vi "Extract TDMS FGEN Info.vi"(8 "error in (no error)":errorcluster, 10 "TDMS Name Mapping":T1, 11 "TDMS File Path":path) -> (0 "error out":errorcluster, 1 "FGEN Sample Rate":dbl, 2 "FGEN Wfm Map":map{string, waveform(dbl)[]}(c390), 3 "FGEN Channels":string[](array[string]), 4 "Gain Per Channel":dbl[](array[numeric]))   [LabVIEW 2025]
uses:
  <vilib>/ErrorRing/Error Ring.xnode
  <vilib>/Utility/error.llb/Error Cluster From Error Code.vi
  Typedef/TDMS Name Mapping.ctl
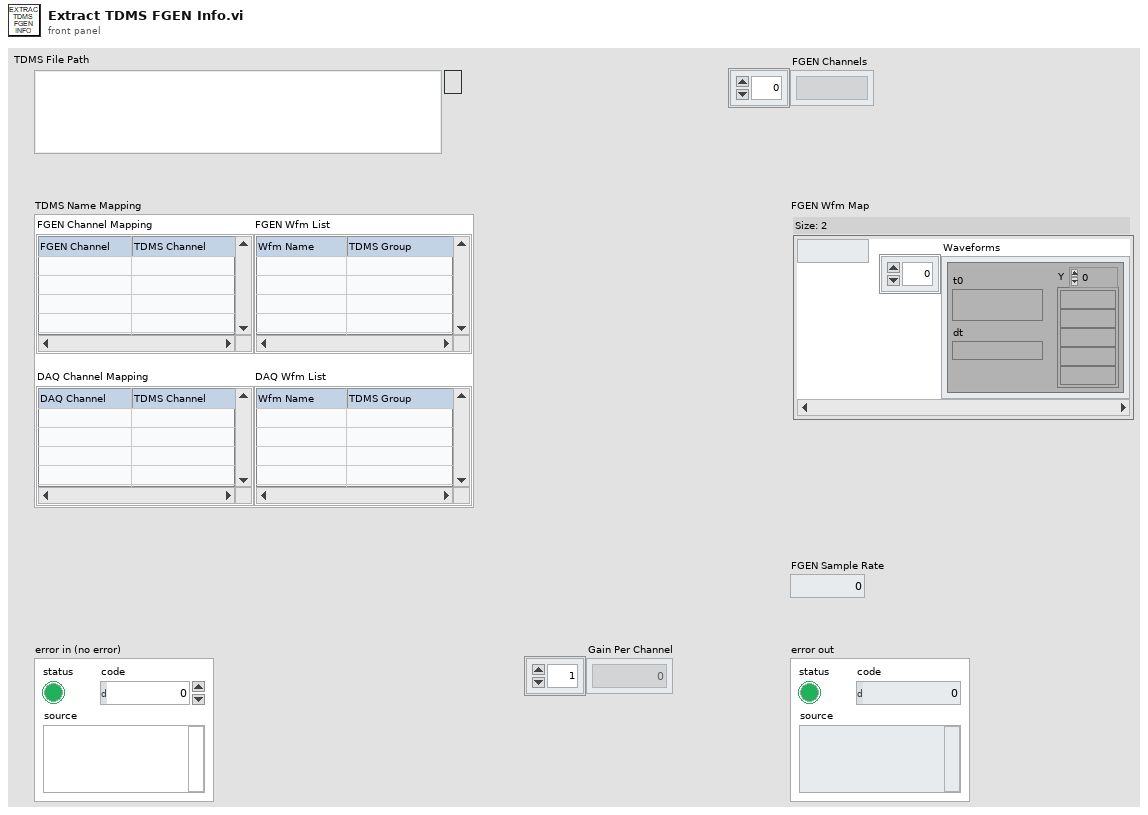
[diagram p1: front panel]
types:
  T1 = typedef "TDMS Name Mapping.ctl" = cluster{"FGEN Channel Mapping":string[][], "DAQ Channel Mapping":string[][], "FGEN Wfm List":string[][], "DAQ Wfm List":string[][]}
  T2 = enum16{"open", "open or create", "create or replace", "create", "open (read-only)"}
  T3 = enum16{"Error or Wfm Not Found", "Not all Chns Found", "All Found"}
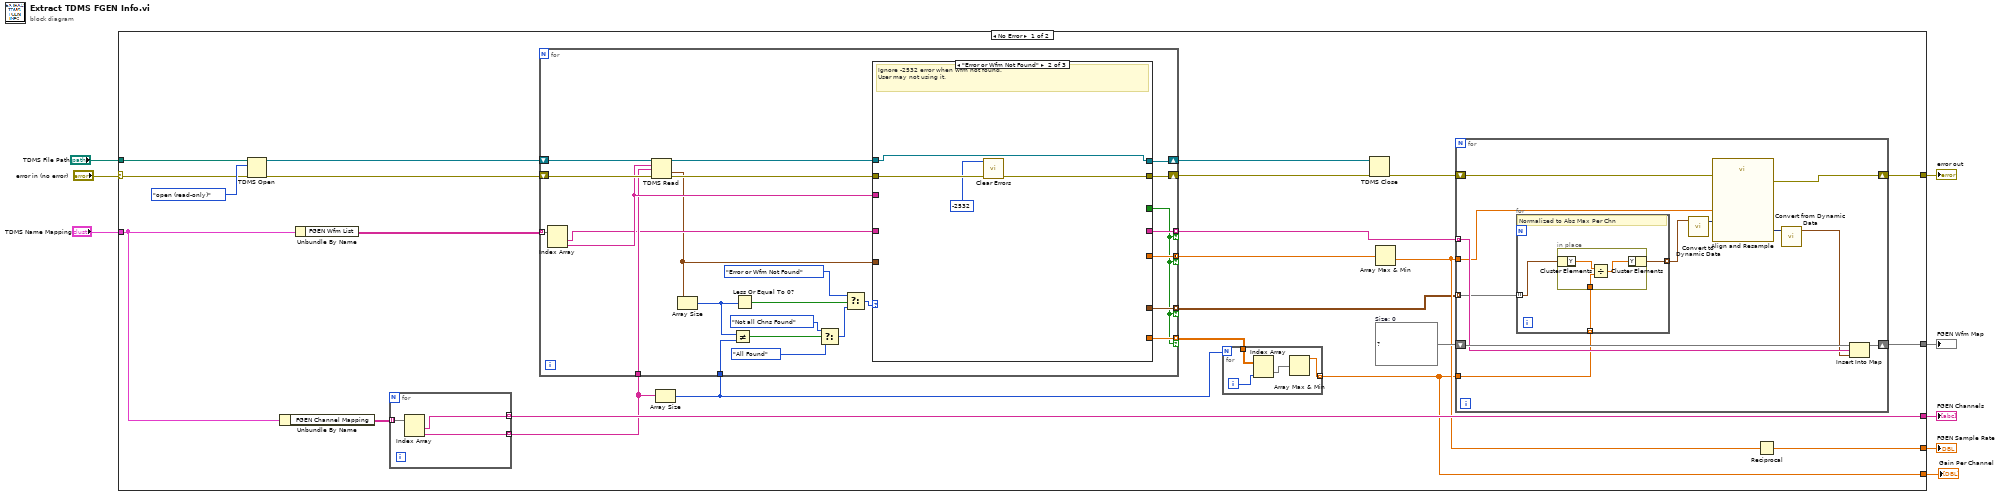
[diagram p0: block diagram]
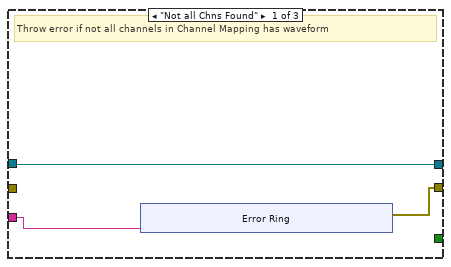
[diagram p2: hidden frame]
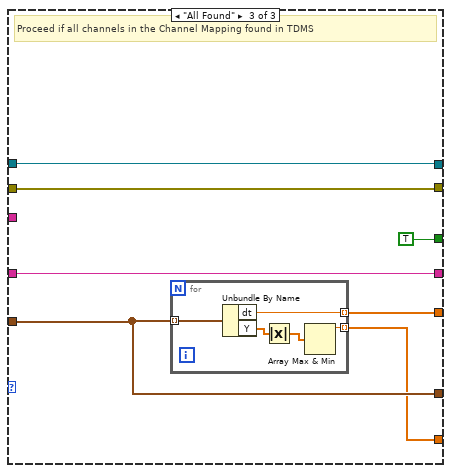
[diagram p3: hidden frame]
diagram:
  n1 = case shown="No Error" "error in (no error)" {
    selector: "error in (no error)" -> [w23 w109]
    tunnel: "TDMS File Path" -> [w30 _]
    tunnel: [w29 _] -> w7
    tunnel: [w18 w109] -> w6
    tunnel: [w17 _] -> w4
    tunnel: [w15 _] -> w3
    tunnel: "TDMS Name Mapping" -> [w13 _]
    tunnel: [w9 _] -> w1
    frame No Error {
      w21 = map{string, waveform(dbl)[]} {}  # Size: 0
      n2 = TDMS Open(8:w23, 10:T2."open (read-only)" ("operation (0:open)"), 11:w30) -> (0:w27:errorcluster, 3:w28:refnum<k34>)  [unwired: 4 in]
      n3 = Unbundle By Name(w13) -> ("FGEN Channel Mapping"=w31:string[][])
      n4 = Unbundle By Name(w13) -> ("FGEN Wfm List"=w32:string[][])
      n5 = for {
        tunnel: w31 -> [w39] mode=indexing
        tunnel: [w38] -> w29 mode=indexing
        tunnel: [w37] -> w14 mode=indexing
        n6 = Index Array(array=w39) -> (element #1=w38:string, element #2=w37:string)  [unwired: 2 in]
      }
      n7 = Array Size(array=w14) -> (size(s)=w10:i32)
      n8 = for {
        tunnel: w32 -> [w64] mode=indexing
        tunnel: [w54] -> w19 mode=indexing if=w40
        tunnel: w14 -> [w56]
        shift-right: [w42] -> w24
        shift-left: w27 -> [w62]
        shift-right: [w60] -> w25
        shift-left: w28 -> [w63]
        tunnel: [w58] -> w12 mode=indexing if=w40
        tunnel: [w57] -> w22 mode=concatenating if=w40
        tunnel: w10 -> [w48]
        tunnel: [w41] -> w11 mode=indexing if=w40
        n9 = Index Array(array=w64) -> (element #1=w55:string, element #2=w59:string)  [unwired: 2 in]
        n10 = TDMS Read(0:w63, 5:w59, 7:w56, 11:w62) -> (4:w61:refnum<k34>, 10:w52:waveform(dbl)[], 15:w53:errorcluster)  [unwired: 4 in, 3 out]
        n11 = Array Size(array=w52) -> (size(s)=w49:i32)
        n12 = Not Equal?(x=w49, y=w48) -> (x != y?=w45:bool)
        n13 = Less Or Equal To 0?(x=w49) -> (x <= 0?=w50:bool)
        n14 = Select(t=T3."Not all Chns Found", s=w45, f=T3."All Found") -> (s? t:f=w46:T3)
        n15 = Select(t=T3."Error or Wfm Not Found", s=w50, f=w46) -> (s? t:f=w43:T3)
        n16 = case shown="\"Error or Wfm Not Found\"" w43 {
          tunnel: w53 -> [_ w77 w85]
          tunnel: w61 -> [w67 w76 w84]
          tunnel: [w67 w76 w84] -> w60
          tunnel: w59 -> [w66 _ _]
          tunnel: [_ _ w80] -> w58
          tunnel: [_ _ w83] -> w57
          tunnel: w52 -> [_ _ w80]
          tunnel: w55 -> [_ _ w82]
          tunnel: [_ _ w82] -> w54
          tunnel: [_ _ TRUE] -> w40
          tunnel: [w65 w78 w85] -> w42
          tunnel: [_ _ w79] -> w41
          frame "Not all Chns Found" {
            # "Throw error if not all channels in Channel Mapping has waveform"
            n17 = xnode "Error Ring"("parameter 0"=w66) -> ("error out"=w65:errorcluster)
          }
          frame "Error or Wfm Not Found" {
            # "Ignore -2532 error when wfm not found.\nUser may not using it."
            n18 = call <vilib>:"Clear Errors.vi"("error in (no error)"=w77, "specific error code to clear (0: all)"=-2532) -> ("error out"=w78:errorcluster)  [unwired: 4 in, 1 out]
          }
          frame "All Found" {
            # "Proceed if all channels in the Channel Mapping found in TDMS"
            n19 = for {
              tunnel: w80 -> [w90] mode=indexing
              tunnel: [w89] -> w83 mode=indexing
              tunnel: [w86] -> w79 mode=indexing
              n20 = Unbundle By Name(w90) -> ("dt"=w89:dbl, "Y"=w88:dbl[])
              n21 = Absolute Value(x=w88) -> (abs(x)=w87:dbl[])
              n22 = Array Max & Min(array=w87) -> (max value=w86:dbl)  [unwired: 3 out]
            }
          }
        }
      }
      n23 = for {
        N: w10 -> [_]
        tunnel: w11 -> [w36]
        tunnel: [w34] -> w9 mode=indexing
        i -> [w33]
        n24 = Index Array(array=w36, index (col)=w33) -> (element=w35:dbl[])  [unwired: 1 in]
        n25 = Array Max & Min(array=w35) -> (max value=w34:dbl)  [unwired: 3 out]
      }
      n26 = TDMS Close(8:w24, 11:w25) -> (0:w20:errorcluster)  [unwired: 1 out]
      n27 = Array Max & Min(array=w22) -> (min value=w16:dbl)  [unwired: 3 out]
      n28 = for {
        tunnel: w12 -> [w94] mode=indexing
        shift-right: [w101] -> w17
        shift-left: w21 -> [w102]
        tunnel: w16 -> [w95]
        shift-right: [w99] -> w18
        shift-left: w20 -> [w100]
        tunnel: w19 -> [w96] mode=indexing
        tunnel: w9 -> [w92]
        n29 = for {
          tunnel: w94 -> [w105] mode=indexing
          tunnel: w92 -> [w104] mode=indexing
          tunnel: [w103] -> w93 mode=indexing
          # "Normalized to Abs Max Per Chn"
          n30 = in-place {
            in-place-border: w104 -> [w107]
            n31 = in-place-cluster #1(w105) -> ("Y"=w108:dbl[])
            n32 = Divide(x=w108, y=w107) -> (x/y=w106:dbl[])
            n33 = in-place-cluster #1("Y"=w106) -> (w103:waveform(dbl))
          }
        }
        n34 = call "Convert to Dynamic Data"("Array of Waveforms"=w93) -> ("Dynamic Data Type"=w98:dynamicdata)  [unwired: 3 in]
        n35 = call "Align and Resample"("dt"=w95, "error in (no error)"=w100, "Signals"=w98) -> ("error out"=w99:errorcluster, "Resampled Signals"=w97:dynamicdata)  [unwired: 6 in, 1 out]
        n36 = call "Convert from Dynamic Data"("Dynamic Data Type"=w97) -> ("Array of Waveform"=w91:waveform(dbl)[])  [unwired: 3 in]
        n37 = Insert Into Map(map in=w102, key=w96, value=w91) -> (map out=w101:map{string, waveform(dbl)[]})  [unwired: 2 out]
      }
      n38 = Reciprocal(x=w16) -> (1/x=w15:dbl)
    }
    frame Error {
    }
  }
  "FGEN Channels" <- w7
  "error out" <- w6
  "FGEN Wfm Map" <- w4
  "FGEN Sample Rate" <- w3
  "Gain Per Channel" <- w1
